vi "MCP4725 Show Computed Values In Graph.vi"() -> ()   [LabVIEW 2014]
uses:
  <vilib>/LabVIEW Universal Transcriptor/LabVIEW for Arduino Math Library/Arduino Math.lvlib
panel:
  out "Waveform Graph 3":i32[](graph)
  in  "Error In":errorcluster
  out "Waveform Graph 2":u16[](graph)
  out "Waveform Graph":i32[](graph)
  out "error IO":errorcluster
  out "Array":i32[](array[numeric])
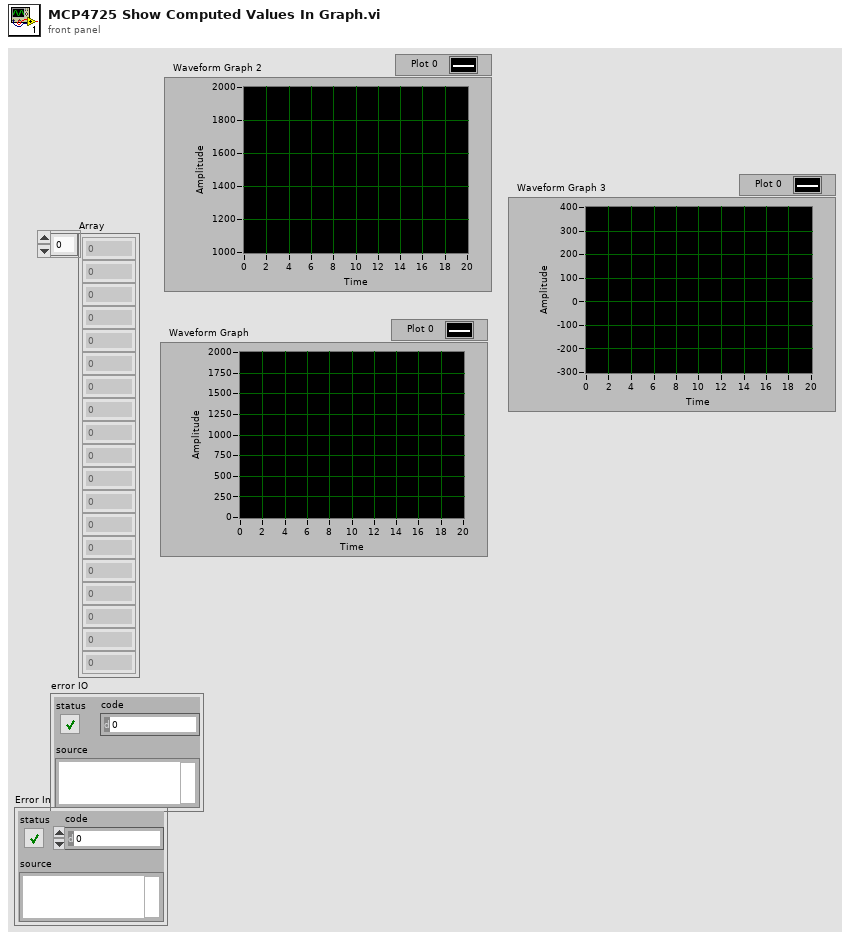
[diagram p1: front panel]
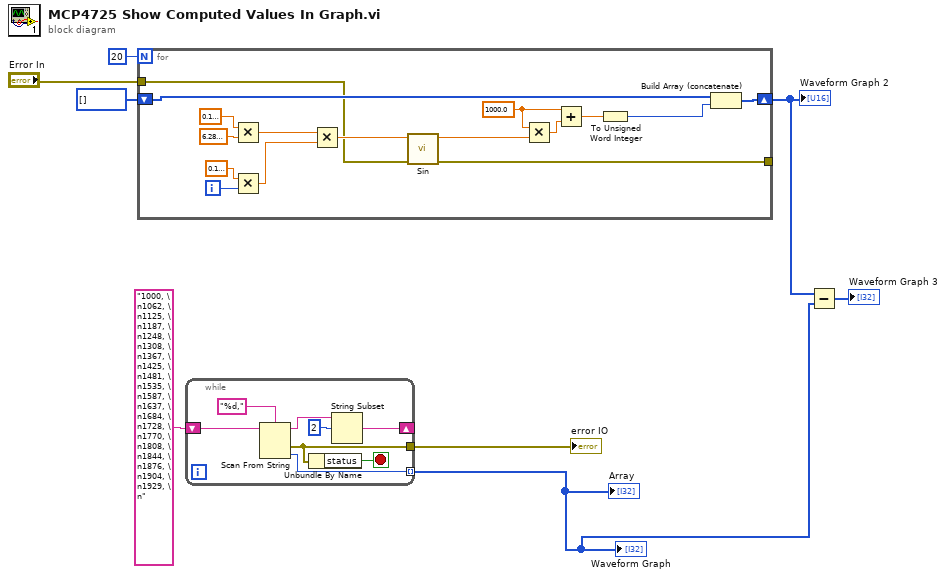
[diagram p0: block diagram]
diagram:
  n1 = for {
    N: 20 -> [_]
    tunnel: [w12] -> _
    shift-right: [w13] -> w3
    shift-left: u16[] [] -> [w14]
    tunnel: "Error In" -> [w9]
    i -> [w21]
    w15 = sgl 1000.0 ("x")
    n2 = Multiply(x=sgl 0.1, y=sgl 6.28 ("x")) -> (x*y=w22:sgl)
    n3 = Multiply(x=sgl 0.1, y=w21) -> (x*y=w19:sgl)
    n4 = Multiply(x=w22, y=w19) -> (x*y=w18:sgl)
    n5 = call <vilib>:"Sin.vi"("Error In"=w9, "x"=w18) -> ("Error Out"=w12:errorcluster, "sin(x)"=w17:sgl)  [unwired: 8 in]
    n6 = Multiply(x=w15, y=w17) -> (x*y=w16:sgl)
    n7 = Add(x=w15, y=w16) -> (x+y=w11:sgl)
    n8 = To Unsigned Word Integer(number=w11) -> (unsigned 16bit integer=w10:u16)
    n9 = Build Array (concatenate)(w14, w10) -> (w13:u16[])
  }
  "Waveform Graph 2" <- w3
  n10 = while {
    shift-right: [w26] -> _
    shift-left: "1000, \n1062, \n1125, \n1187, \n1248, \n1308, \n1367, \n1425, \n1481, \n1535, \n1587, \n1637, \n1684, \n1728, \n1770, \n1808, \n1844, \n1876, \n1904, \n1929, \n" -> [w31]
    tunnel: [w30] -> w2 mode=indexing
    tunnel: [w25] -> w7
    stop <- w29 stop-if-true
    n11 = Scan From String(format string="%d,", input string=w31) -> (remaining string=w28:string, error out=w25:errorcluster, output 1=w30:i32)  [unwired: 3 in, 1 out]
    n12 = Unbundle By Name(w25) -> ("status"=w29:bool)
    n13 = String Subset(string=w28, offset (0)=2) -> (substring=w26:string)  [unwired: 1 in]
  }
  "Array" <- w2
  "error IO" <- w7
  "Waveform Graph" <- w2
  n14 = Subtract(x=w3, y=w2) -> (x-y=→"Waveform Graph 3":i32[])
